vi "Init Output.vi"(8 "error in (no error)":errorcluster, 10 "Descriptor":string, 11 "output in":refnum<class "Output.lvclass">) -> (0 "error out":errorcluster, 3 "output out":refnum<class "Output.lvclass">)   [LabVIEW 2015, in "Output.lvclass"]
uses:
  Output.lvclass
  Output.lvclass/Output.ctl
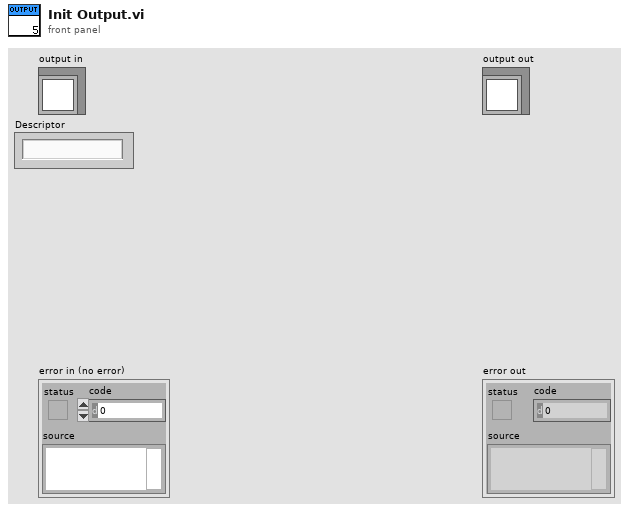
[diagram p1: front panel]
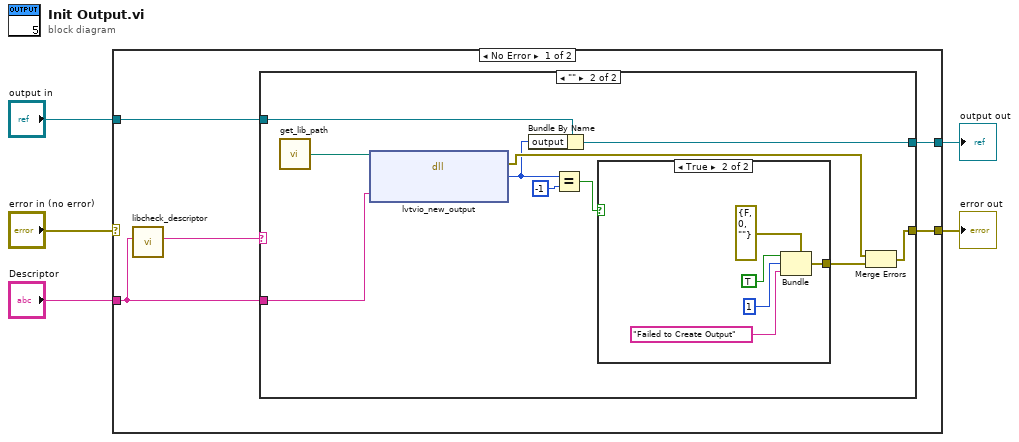
[diagram p0: block diagram]
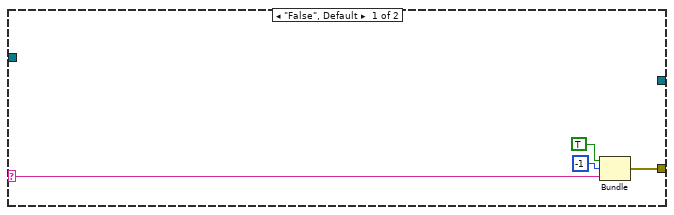
[diagram p2: hidden frame]
diagram:
  n1 = case shown="No Error" "error in (no error)" {
    selector: "error in (no error)" -> [_ w31]
    tunnel: [w7 w31] -> w4
    tunnel: [w8 w30] -> w2
    tunnel: "output in" -> [w6 w30]
    tunnel: "Descriptor" -> [w9 _]
    frame No Error {
      n2 = call "libcheck_descriptor.vi"("Descriptor"=w9) -> ("result"=w10:string)  [unwired: 9 in, 1 out]
      n3 = case shown="\"\"" w10 {
        selector: w10 -> [w12 _]
        tunnel: [_ w18] -> w8
        tunnel: [w11 w17] -> w7
        tunnel: w9 -> [_ w16]
        tunnel: w6 -> [_ w15]
        frame "False", Default {
          n4 = Bundle("status"=TRUE, "code"=-1, w12) -> (w11:cluster{"status":bool, "code":i32, string})  [unwired: 1 in]
        }
        frame "" {
          n5 = call "get_lib_path.vi"() -> ("Path"=w24:path)
          n6 = dll-call lib="S:/thingiverselv/lib/liblvtvio.dll" fn="lvtvio_new_output"(path in=w24, "descriptor"=w16) -> (error out=w20:errorcluster, "return type"=w19:i32)  [unwired: 3 in, 1 out]
          n7 = Bundle By Name(cluster=w15, "output"=w19) -> (w18:refnum<class "Output.lvclass">)
          n8 = Equal?(x=w19, y=-1) -> (x = y?=w22:bool)
          n9 = case shown="True" w22 {
            tunnel: [_ w25] -> w21
            frame False {
            }
            frame True {
              n10 = Bundle(cluster=errorcluster {"status"=FALSE, "code"=0, "source"=""} ("error in (no error)"), "status"=TRUE, "code"=1, "source"="Failed to Create Output") -> (w25:errorcluster)
            }
          }
          n11 = Merge Errors(w20, w21) -> (w17:errorcluster)
        }
      }
    }
    frame Error {
    }
  }
  "error out" <- w4
  "output out" <- w2
